vi "NI VeriStand - Wait on FPGA Clock.vi"() -> (0 "Clock Ticked":bool)   [LabVIEW 2010, in "NI_VS FPGA Clock Support.lvlib"]
uses:
  <userlib>/_NI VeriStand FPGA Support/NI VeriStand FPGA Clock Support/NI_VS FPGA Clock Support.lvlib
  <vilib>/Platform/TimedLoop/XDataNode/XDataNode.xnode
  <vilib>/Platform/TimedLoop/XDataNode/timing_clust.ctl
  <vilib>/Platform/TimedLoop/XDataNode/nitl_modes.ctl
  <vilib>/Platform/TimedLoop/XDataNode/wakeup.ctl
  <userlib>/_NI VeriStand FPGA Support/NI VeriStand FPGA Clock Support/NI VeriStand - Timing Engine Globals.vi
  <vilib>/Platform/TimedLoop/XDataNode/XDNodeRunTimeDep.lvlib
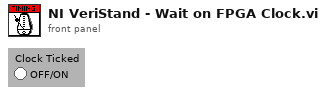
[diagram p1: front panel]
types:
  T1 = typedef "XDNodeRunTimeDep.lvlib/timing_clust.ctl" = cluster{"Expected End [f-1]":u64, "Actual End [f-1]":u64, "Finished Late? [f-1]":bool, "Expected End [i-1]":u64, "Actual End [i-1]":u64, "Finished Late? [i-1]":bool, "Expected Start [i]":u64, "Actual Start [i]":u64, "Expected Start [f]":u64, "Actual Start [f]":u64, "Source Name":string, "Structure Name":string, "Period":i64, "Deadline":i64, "Offset":i64, "Start":i64, "Priority":i32, "Timeout":i32, "Mode":T2, "Wakeup Reason":T3, "Error":errorcluster, "Source Type":string, "Secondary Source Type":string, "Global End Time":u64, "Global Start Time":u64, "Frame Duration":u64, "Iteration Duration":u64, "Assigned CPU":i32, "I/O Scan Engine Mode":u32}
  T2 = typedef "XDNodeRunTimeDep.lvlib/nitl_modes.ctl" = enum32{"No Change", "Process missed periods, maintain original phase", "Discard missed periods, maintain original phase", "Process missed periods, ignore original phase", "Discard missed periods, ignore original phase"}
  T3 = typedef "XDNodeRunTimeDep.lvlib/wakeup.ctl" = enum32{"Normal", "Aborted", "Asynchronous wakeup", "Timing source error", "Timed loop error", "Timeout"}
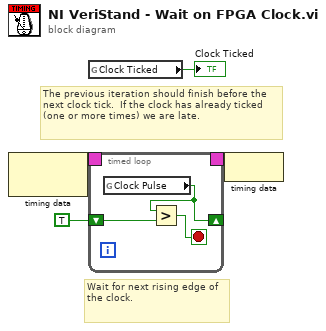
[diagram p0: block diagram]
diagram:
  # "The previous iteration should finish before the next clock tick.  If the clock has already ticked (one or more times) we are late."
  # "Wait for next rising edge of the clock."
  n1 = node-c288() -> (w4:T1)  [unwired: 1 out]
  n2 = global read "NI VeriStand - Timing Engine Globals.vi" "Clock Ticked"() -> (→"Clock Ticked":bool)
  n3 = timed-loop {
    timing: w4 -> [_]
    timing-out: [_] -> w3
    shift-right: [w5] -> _
    shift-left: TRUE ("Clock Ticked") -> [w7]
    stop <- w6 stop-if-true
    n4 = global read "NI VeriStand - Timing Engine Globals.vi" "Clock Pulse"() -> (w5:bool)
    n5 = Greater?(x=w5, y=w7) -> (0:w6:bool)
  }
  n6 = node-c288(w3) -> ()
